vi "Write Shared Variables.vi"(10 "Read Values":dbl[](array[numeric]), 11 "Shared Variables to Write in":T1) -> (0 "error out":errorcluster, 3 "Shared Variables to Write out":T1)   [LabVIEW 2012, in "Shared Variable Custom Device.lvlib"]
uses:
  Shared Variable Custom Device.lvlib
  Shared Variable/Shared Variable Cluster.ctl
  Shared Variable/Shared Variable Access.ctl
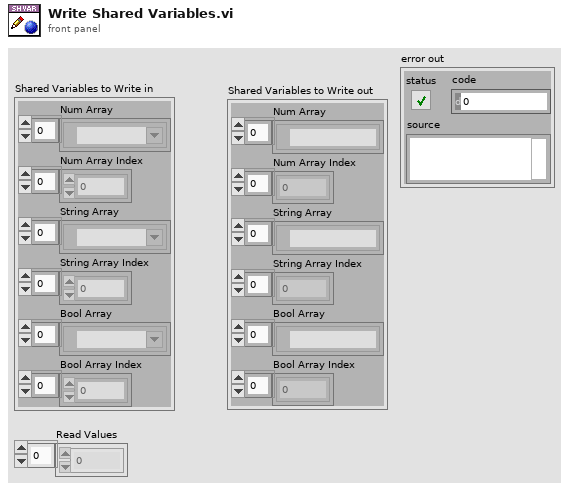
[diagram p1: front panel]
types:
  T1 = typedef "Shared Variable Custom Device.lvlib/Shared Variable Cluster.ctl" = cluster{"Num Array":refnum<k21>[], "Num Array Index":i32[], "String Array":refnum<k21>[], "String Array Index":i32[], "Bool Array":refnum<k21>[], "Bool Array Index":i32[]}
  T2 = typedef "Shared Variable Custom Device.lvlib/Shared Variable Access.ctl" = enum16{"Write", "Read"}
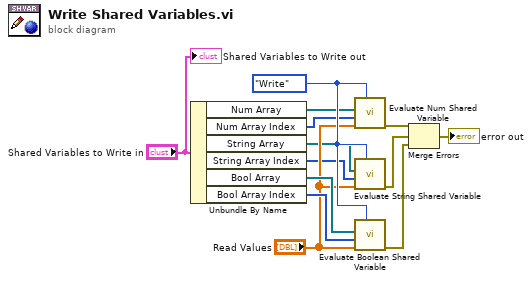
[diagram p0: block diagram]
diagram:
  w13 = Shared_Variable_Access."Write" ("Access")
  n1 = Unbundle By Name("Shared Variables to Write in") -> ("Num Array"=w6:refnum<k21>[], "Num Array Index"=w7:i32[], "String Array"=w8:refnum<k21>[], "String Array Index"=w9:i32[], "Bool Array"=w11:refnum<k21>[], "Bool Array Index"=w12:i32[])
  n2 = call "Evaluate Num Shared Variable.vi"("Access"=w13, "Read Values"="Read Values", "Num Array Index"=w7, "Num Array"=w6) -> ("error out"=w4:errorcluster)  [unwired: 6 in, 1 out]
  n3 = call "Evaluate String Shared Variable.vi"("Access"=w13, "Read Values"="Read Values", "String Array Index"=w9, "String Array"=w8) -> ("error out"=w3:errorcluster)  [unwired: 6 in, 1 out]
  n4 = call "Evaluate Boolean Shared Variable.vi"("Access"=w13, "Read Values"="Read Values", "Boolean Array Index"=w12, "Boolean Array"=w11) -> ("error out"=w2:errorcluster)  [unwired: 6 in, 1 out]
  n5 = Merge Errors(w4, w3, w2) -> (→"error out":errorcluster)
  "Shared Variables to Write out" <- "Shared Variables to Write in"
